vi "serial read v2.vi"() -> ()   [LabVIEW 2023]
uses:
  <vilib>/Instr/_visa.llb/VISA Configure Serial Port (Instr).vi
panel:
  out "return count":u32
  out "concatenated string":string
  in  "Slide 2":dbl(slide) scale=0.0..1000.0
  in  "write buffer":string
  in  "baud rate (9600)":u32=9600
  out "read buffer":string
  out "Loop Number":i32
  in  "stop":bool
  in  "COM":refnum<visa-resource-name>
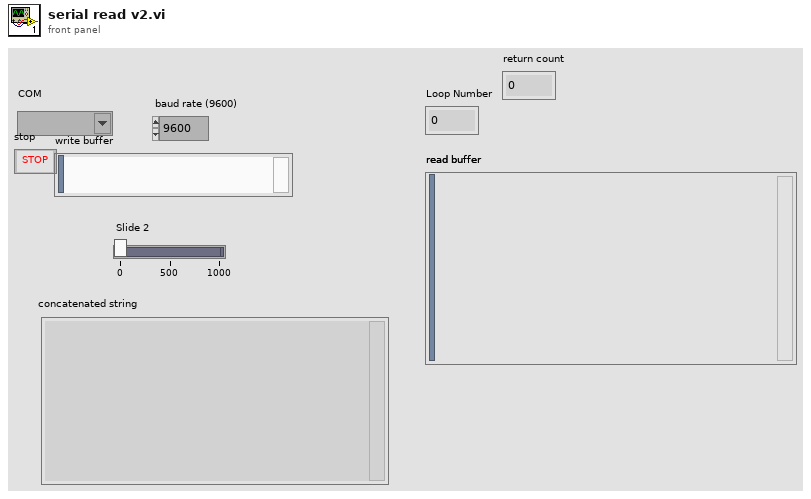
[diagram p1: front panel]
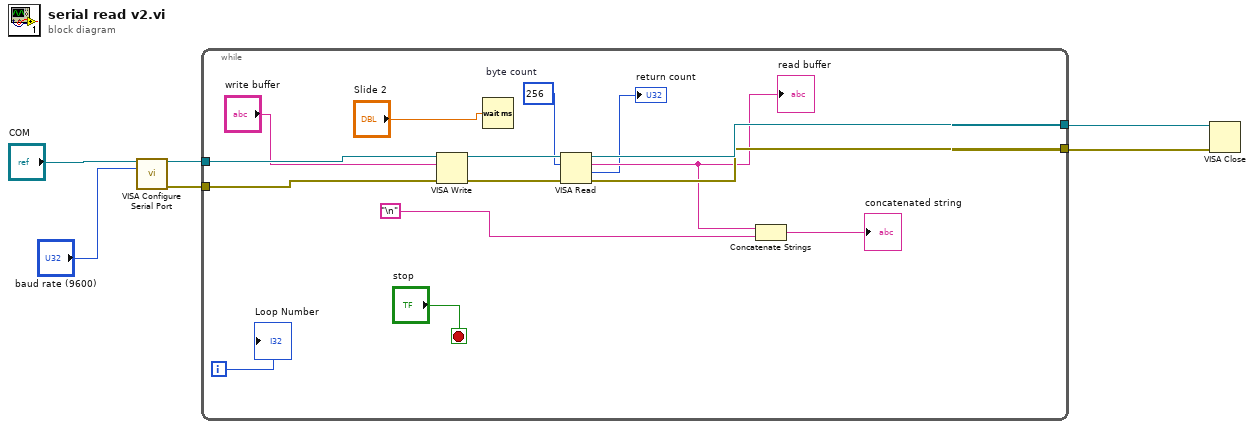
[diagram p0: block diagram]
diagram:
  n1 = call-poly "VISA Configure Serial Port"("VISA resource name"="COM", "baud rate (9600)"="baud rate (9600)") -> ("VISA resource name out"=w5:refnum<visa-resource-name>, "error out"=w6:errorcluster)  [unwired: 12 in]
  n2 = while {
    tunnel: w6 -> [w18]
    tunnel: w5 -> [w19]
    tunnel: [w17] -> w2
    tunnel: [w16] -> w1
    i -> [w20]
    stop <- "stop" stop-if-true
    w12 = u32 256  # byte count
    n3 = VISA Write(VISA resource name=w19, write buffer="write buffer", error in (no error)=w18) -> (VISA resource name out=w13:refnum<visa-resource-name>, error out=w11:errorcluster)  [unwired: 1 out]
    n4 = Wait (ms)(milliseconds to wait="Slide 2") -> ()  [unwired: 1 out]
    n5 = VISA Read(VISA resource name=w13, byte count=w12, error in (no error)=w11) -> (VISA resource name out=w17:refnum<visa-resource-name>, read buffer=w9:string, return count=→"return count":u32, error out=w16:errorcluster)
    "read buffer" <- w9
    n6 = Concatenate Strings(w9, "\n") -> (→"concatenated string":string)
    "Loop Number" <- w20
  }
  n7 = VISA Close(VISA resource name=w2, error in (no error)=w1) -> ()  [unwired: 1 out]
